vi "Write ModulePath.vi"(8 "error in (no error)":errorcluster, 10 "ModulePath":path, 11 "PythonWrapper in":refnum<class "PythonWrapper.lvclass">) -> (0 "error out":errorcluster, 3 "PythonWrapper out":refnum<class "PythonWrapper.lvclass">)   [LabVIEW 2022 SP3, in "PythonWrapper.lvlib" / "PythonWrapper.lvclass"]
uses:
  PythonWrapper.lvclass
  PythonWrapper.lvclass/PythonWrapper.ctl
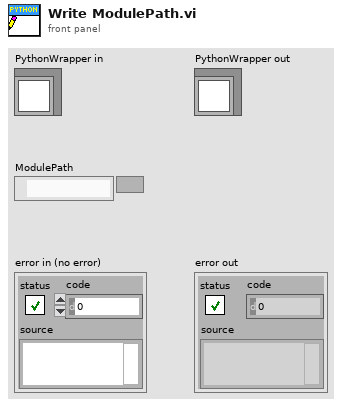
[diagram p1: front panel]
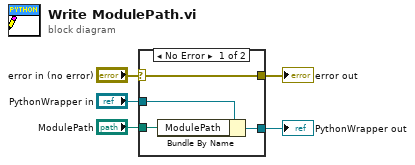
[diagram p0: block diagram]
diagram:
  n1 = case shown="No Error" "error in (no error)" {
    selector: "error in (no error)" -> [w9 w10]
    tunnel: [w9 w10] -> w4
    tunnel: [w7 w11] -> w2
    tunnel: "PythonWrapper in" -> [w8 w11]
    tunnel: "ModulePath" -> [w6 _]
    frame No Error {
      n2 = Bundle By Name(cluster=w8, "ModulePath"=w6) -> (w7:refnum<class "PythonWrapper.lvclass">)
    }
    frame Error {
    }
  }
  "error out" <- w4
  "PythonWrapper out" <- w2
